vi "Visit Me.vi"(8 "error in (no error)":errorcluster, 10 "Visitor In":refnum<class "LVTypeVisitor.lvclass">, 11 "LVType in":refnum<class "LVType.lvclass">) -> (0 "error out":errorcluster, 2 "Visitor Out":refnum<class "LVTypeVisitor.lvclass">, 3 "LVType out":refnum<class "LVType.lvclass">)   [LabVIEW 2020, in "LVDataTypes.lvlib" / "LVType.lvclass"]
uses:
  <vilib>/AppBuilder/Engine/WebServiceDescription/LVDataTypes/LVType/LVType.lvclass
  <vilib>/AppBuilder/Engine/WebServiceDescription/LVDataTypes/LVTypeVisitor/LVTypeVisitor.lvclass
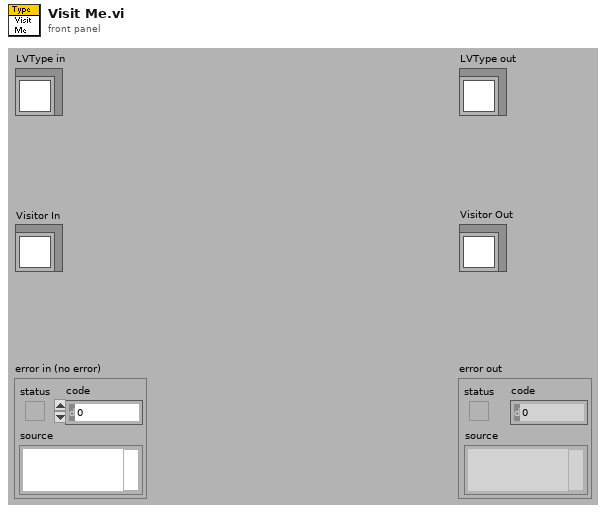
[diagram p1: front panel]
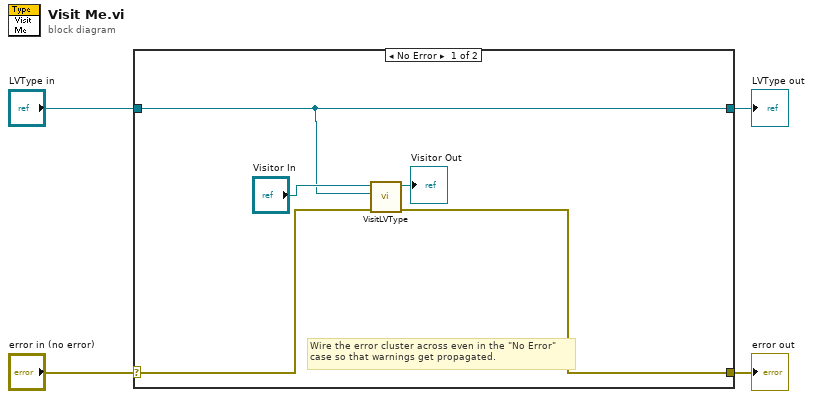
[diagram p0: block diagram]
diagram:
  n1 = case shown="No Error" "error in (no error)" {
    selector: "error in (no error)" -> [w6 w11]
    tunnel: [w5 w11] -> w3
    tunnel: [w8 w10] -> w1
    tunnel: "LVType in" -> [w8 w10]
    frame No Error {
      # "Wire the error cluster across even in the \"No Error\"\ncase so that warnings get propagated."
      n2 = call-dynamic "VisitLVType.vi"("error in (no error)"=w6, "LVType"=w8, "LVTypeVisitor in"="Visitor In") -> ("error out"=w5:errorcluster, "LVTypeVisitor out"=→"Visitor Out":refnum<class "LVTypeVisitor.lvclass">)  [unwired: 7 out]
    }
    frame Error {
    }
  }
  "error out" <- w3
  "LVType out" <- w1
